vi "Main.vi"() -> ()   [LabVIEW 2013]
uses:
  <vilib>/Analysis/Matrix/Datatypes/RealMatrix.ctl
  Parts.ctl
  ROS/Code/SubVIs/BaxterSide.ctl
  ROS/Code/SubVIs/BaxterCamera.ctl
  Arm Globals.vi
  Prim/Fwd Kenimatics - array.vi
  Move/Move Axis.vi
  Move/Move XYZOAT.vi
  <vilib>/Analysis/Matrix/NI_Matrix.lvlib
panel:
  in  "To":string="Table"
  in  "From":string="Table"
  in  "Both?":bool
  in  "Post Side":bool
  in  "Side":T1=enum."right"
  in  "Go Via":bool
  in  "Increment":dbl=50.0
  in  "Offset":cluster{"x":dbl, "y":dbl, "a":dbl}={"x"=50.0, "y"=900.0, "a"=0.0}
  in  "Offset":cluster{"x":dbl, "y":dbl, "a":dbl}={"x"=50.0, "y"=900.0, "a"=0.0}
  in  "Put":bool
  in  "Locate Tray":bool
  in  "Part":T2 items=["Big_Gear", "Medium_Gear", "Small_Gear", "Bottom_Cover", "Top_Cover"]
  in  "Fetch":bool
  out "T":T3=[[0.016284994521607307, 0.9998576764567041, 0.0044074691186384496, -12.095922523672678], [0.9998670931969393, -0.01628143110047913, -0.0008431744914288715, -1019.3924117975101], [-0.0007712945830650122, 0.004420614427981981, -0.999989931585686, 240.25900755427352], [0.0, 0.0, 0.0, 1.0]] format="%.3f"
  out "picture":picture
  out "Range":u32=104
  in  "Speed":dbl=25.0
  in  "Shift":cluster{"x":dbl, "y":dbl, "a":dbl}={"x"=-110.0, "y"=-70.0, "a"=0.0}
  in  "Shift":bool
  in  "Go Safe":bool
  in  "Save Pic":bool
  in  "Image":bool
  in  "Gripper":bool caption="Open\n\n\n\nClose"
  in  "Hover Height":dbl=200.0
  in  "Hover":bool
  # "Y"
  # "X"
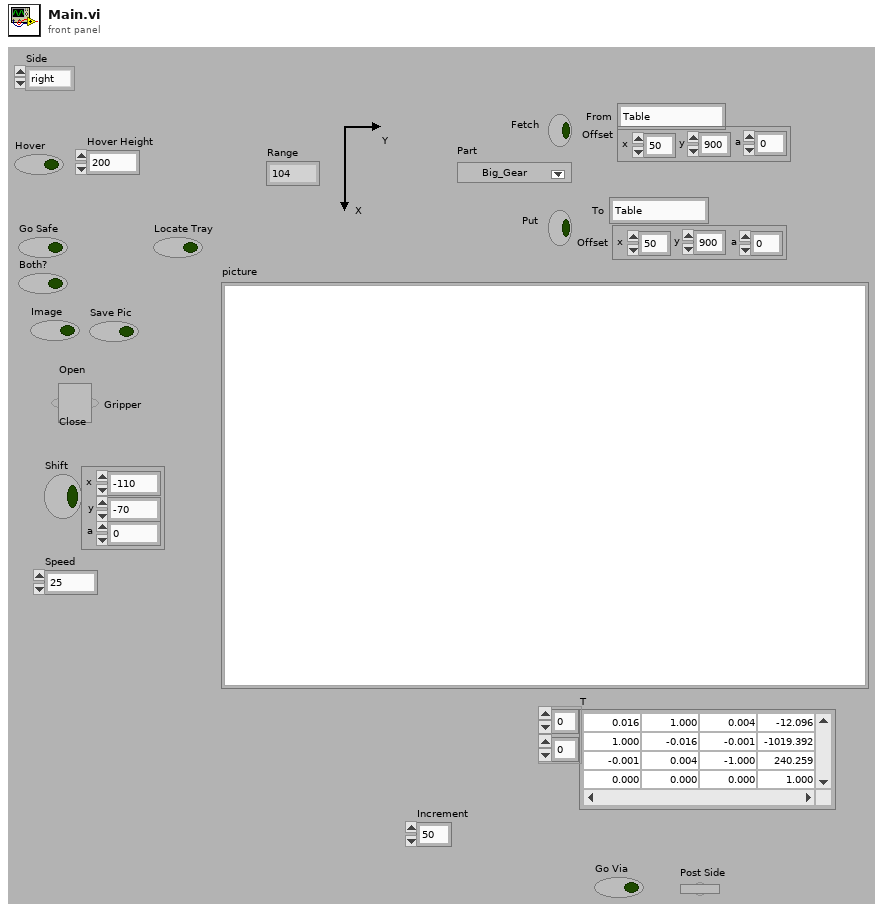
[diagram p1: front panel]
types:
  T1 = typedef "BaxterSide.ctl" = enum16{"left", "right"}
  T2 = typedef "Parts.ctl" = u16
  T3 = typedef "NI_Matrix.lvlib/RealMatrix.ctl" = dbl[][]
  T4 = typedef "BaxterCamera.ctl" = enum16{"left_hand_camera", "right_hand_camera", "head_camera"}
  T5 = cluster{"X":dbl, "Y":dbl, "Z":dbl, "Roll":dbl, "Pitch":dbl, "Yaw":dbl}
  T6 = typedef "imagedata.ctl" = cluster{"image type":i32, "image depth":i32, "image":u8[], "mask":u8[], "colors":u32[], "Rectangle":cluster{"left":i16, "top":i16, "right":i16, "bottom":i16}}
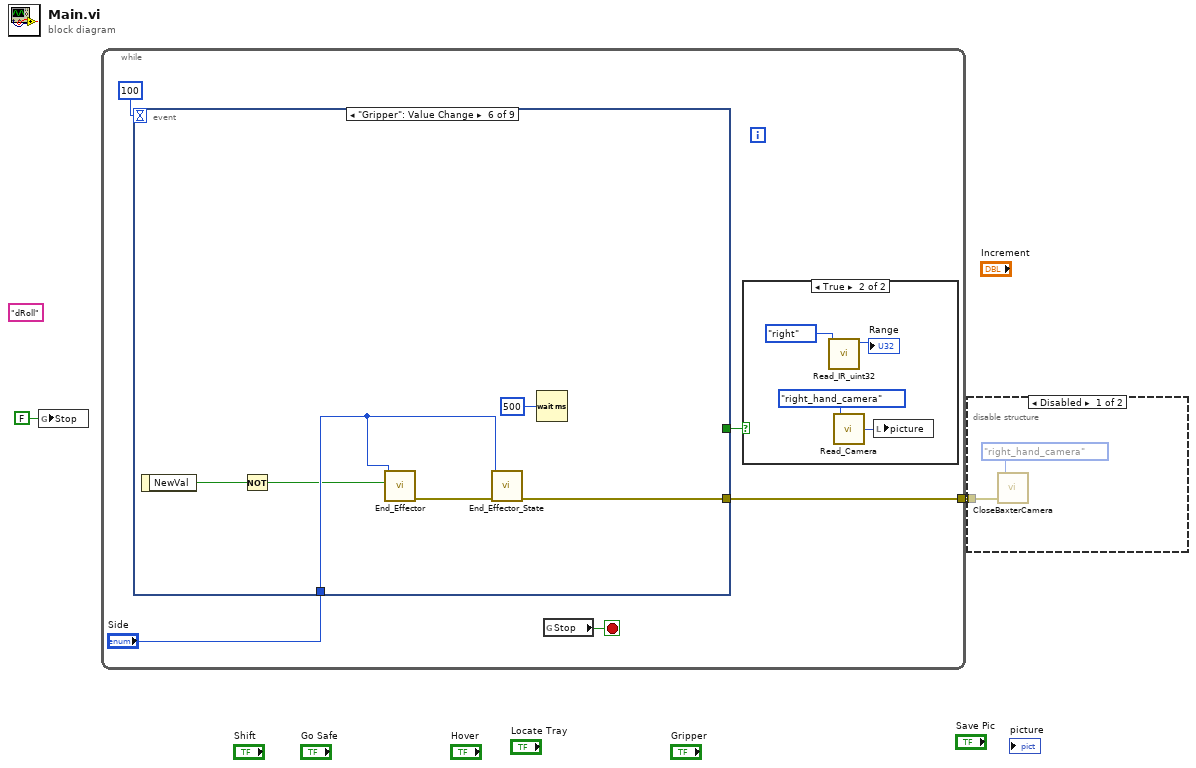
[diagram p0: block diagram]
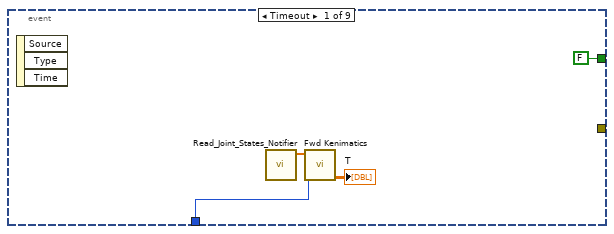
[diagram p4: hidden frame]
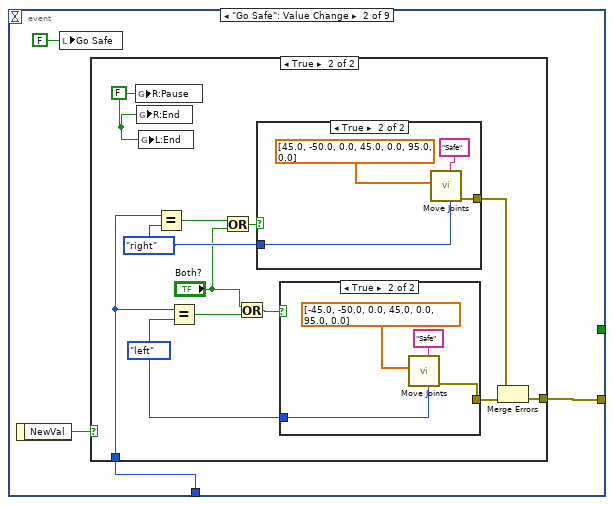
[diagram p5: hidden frame]
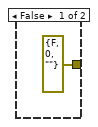
[diagram p6: hidden frame]
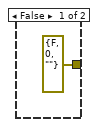
[diagram p7: hidden frame]
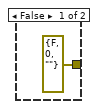
[diagram p8: hidden frame]
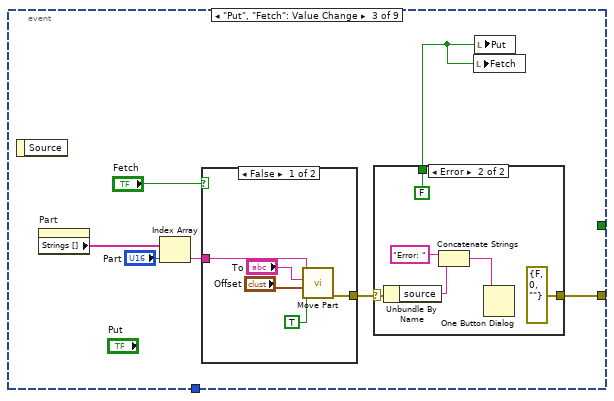
[diagram p9: hidden frame]
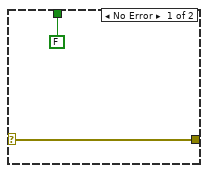
[diagram p10: hidden frame]
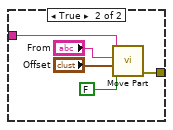
[diagram p11: hidden frame]
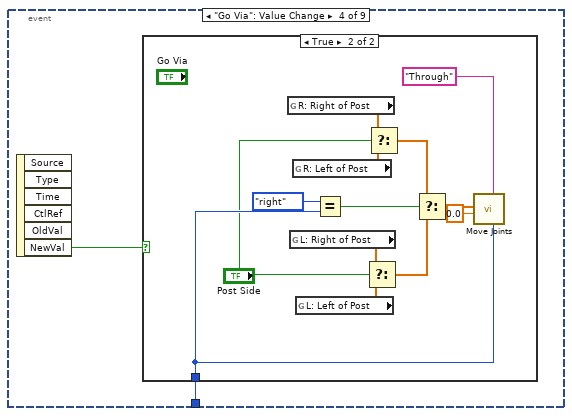
[diagram p12: hidden frame]
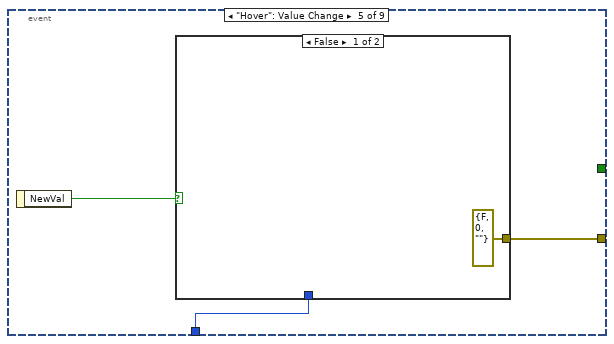
[diagram p14: hidden frame]
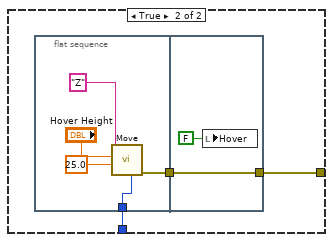
[diagram p15: hidden frame]
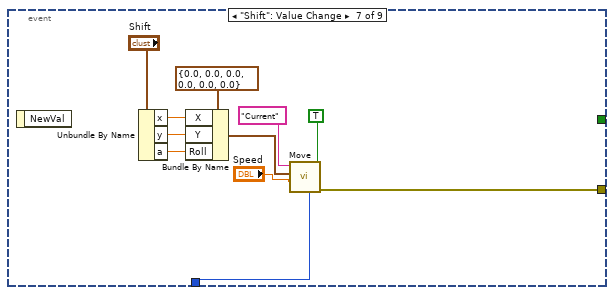
[diagram p16: hidden frame]
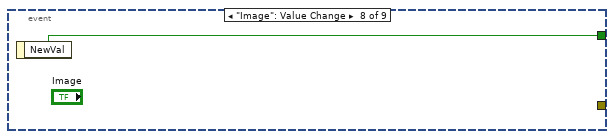
[diagram p17: hidden frame]
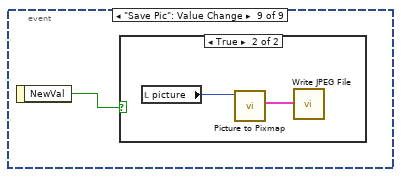
[diagram p18: hidden frame]
diagram:
  (unwired) "dRoll" ("Label")
  n1 = global write "Arm Globals.vi" "Stop"(FALSE ("Stop")) -> ()
  n2 = while {
    tunnel: [w6] -> w1
    stop <- w7 stop-if-true
    n3 = event shown="[5] \"Gripper\": Value Change" {
      selector: _ -> [_ _ _ _ _ _ _ _ _]
      dyn-events: _ -> [_ _ _ _ _ _ _ _ _]
      timeout: 100 -> [_ _ _ _ _ _ _ _ _]
      tunnel: [_ w18 w43 _ w84 w99 w113 _ _] -> w6
      tunnel: "Side" -> [w13 w16 _ w68 w83 w98 w103 _ _]
      tunnel: [FALSE ("NewVal") _ _ _ _ _ _ w114 _] -> w4
      event Timeout {
        n4 = event-data() -> ()  [unwired: 1 in, 3 out]
        n5 = call "Read_Joint_States_Notifier.vi"() -> ("Positions"=w14:dbl[])  [unwired: 7 in, 1 out]
        n6 = call-poly "Fwd Kenimatics.vi"("Side"=w13, "Joints"=w14) -> ("Matrix"=→"T":T3)  [unwired: 8 in, 1 out]
      }
      event "Go Safe": Value Change {
        n7 = event-data() -> ("NewVal"=w19:bool)  [unwired: 1 in]
        n8 = local write "Go Safe"(FALSE ("Go Safe")) -> ()
        n9 = case shown="True" w19 {
          tunnel: [errorcluster {"status"=FALSE, "code"=0, "source"=""} ("error IO") w32] -> w18
          tunnel: w16 -> [_ w28]
          frame False {
          }
          frame True {
            w27 = BaxterSide."left" ("x")
            w29 = BaxterSide."right" ("x")
            w21 = FALSE ("R:Pause")
            n10 = global write "Arm Globals.vi" "R:Pause"(w21) -> ()
            n11 = global write "Arm Globals.vi" "R:End"(w21) -> ()
            n12 = global write "Arm Globals.vi" "L:End"(w21) -> ()
            n13 = Equal?(x=w28, y=w29) -> (x = y?=w23:bool)
            n14 = Equal?(x=w28, y=w27) -> (x = y?=w24:bool)
            n15 = Or(x=w23, y="Both?") -> (x .or. y?=w26:bool)
            n16 = Or(x="Both?", y=w24) -> (x .or. y?=w25:bool)
            n17 = case shown="True" w26 {
              tunnel: w29 -> [_ w36]
              tunnel: [errorcluster {"status"=FALSE, "code"=0, "source"=""} ("error out") w35] -> w30
              frame False {
              }
              frame True {
                n18 = call "Move Joints.vi"("Side"=w36, "Label"="Safe", "Goal"=dbl[] [45.0, -50.0, 0.0, 45.0, 0.0, 95.0, 0.0] ("Joints")) -> ("error out"=w35:errorcluster)  [unwired: 7 in, 1 out]
              }
            }
            n19 = case shown="True" w25 {
              tunnel: [errorcluster {"status"=FALSE, "code"=0, "source"=""} ("error out") w40] -> w31
              tunnel: w27 -> [_ w39]
              frame False {
              }
              frame True {
                n20 = call "Move Joints.vi"("Side"=w39, "Label"="Safe", "Goal"=dbl[] [-45.0, -50.0, 0.0, 45.0, 0.0, 95.0, 0.0] ("Joints")) -> ("error out"=w40:errorcluster)  [unwired: 7 in, 1 out]
              }
            }
            n21 = Merge Errors(w30, w31) -> (w32:errorcluster)
          }
        }
      }
      event "Put", "Fetch": Value Change {
        n22 = event-data() -> ()  [unwired: 1 in, 1 out]
        n23 = property on="Part" class="Ring (strict)"() -> ("Strings []"=w47:string[])  [unwired: 2 in, 2 out]
        n24 = Index Array(array=w47, index="Part") -> (element=w48:string)
        n25 = case shown="False" "Fetch" {
          tunnel: [w62 w67] -> w45
          tunnel: w48 -> [w59 w64]
          frame False {
            n26 = call "Move Part.vi"("Place"=TRUE ("Place?"), "Offset"="Offset", "Location"="To", "Part Name"=w59) -> ("error out"=w62:errorcluster)  [unwired: 7 in]
          }
          frame True {
            n27 = call "Move Part.vi"("Place"=FALSE ("Place?"), "Offset"="Offset", "Location"="From", "Part Name"=w64) -> ("error out"=w67:errorcluster)  [unwired: 7 in]
          }
        }
        n28 = case shown="Error" w45 {
          selector: w45 -> [w50 w56]
          tunnel: [FALSE ("Compute Pose") FALSE ("Compute Pose")] -> w44
          tunnel: [w50 errorcluster {"status"=FALSE, "code"=0, "source"=""} ("error IO")] -> w43
          frame No Error {
          }
          frame Error {
            n29 = Unbundle By Name(w56) -> ("source"=w54:string)
            n30 = Concatenate Strings("Error: " ("string"), w54) -> (w53:string)
            n31 = One Button Dialog(message=w53) -> ()  [unwired: 1 in, 1 out]
          }
        }
        n32 = local write "Fetch"(w44) -> ()
        n33 = local write "Put"(w44) -> ()
      }
      event "Go Via": Value Change {
        n34 = event-data() -> ("NewVal"=w69:bool)  [unwired: 1 in, 5 out]
        n35 = case shown="True" w69 {
          tunnel: w68 -> [_ w77]
          frame False {
          }
          frame True {
            n36 = global read "Arm Globals.vi" "R: Right of Post"() -> (w70:dbl[])
            n37 = global read "Arm Globals.vi" "L: Right of Post"() -> (w75:dbl[])
            n38 = global read "Arm Globals.vi" "R: Left of Post"() -> (w72:dbl[])
            n39 = global read "Arm Globals.vi" "L: Left of Post"() -> (w74:dbl[])
            n40 = Equal?(x=BaxterSide."right", y=w77) -> (x = y?=w80:bool)
            n41 = Select(t=w75, s="Post Side", f=w74) -> (s? t:f=w76:dbl[])
            n42 = Select(t=w70, s="Post Side", f=w72) -> (s? t:f=w73:dbl[])
            n43 = Select(t=w73, s=w80, f=w76) -> (s? t:f=w78:dbl[])
            n44 = call "Move Joints.vi"("Side"=w77, "Label"="Through" ("format string"), "time"=0.0, "Goal"=w78) -> ()  [unwired: 6 in, 2 out]
          }
        }
      }
      event "Hover": Value Change {
        n45 = event-data() -> ("NewVal"=w85:bool)  [unwired: 1 in]
        n46 = case "Move to High Hover" shown="False" w85 {
          tunnel: [errorcluster {"status"=FALSE, "code"=0, "source"=""} ("error out") w89] -> w84
          tunnel: w83 -> [_ w88]
          frame False {
          }
          frame True {
            n47 = flat-sequence {
              tunnel: w88 -> [w90]
              tunnel: [w94] -> w87
              tunnel: [w96] -> w89
              tunnel: w87 -> [w96]
              frame #0 {
                n48 = call-poly "Move.vi"("Side"=w90, "Speed"=25.0, "Value"="Hover Height", "Location"="Z" ("Axis")) -> ("error out"=w94:errorcluster)  [unwired: 7 in]
              }
              frame #1 {
                n49 = local write "Hover"(FALSE ("Hover")) -> ()
              }
            }
          }
        }
      }
      event "Gripper": Value Change {
        n50 = event-data() -> ("NewVal"=w102:bool)  [unwired: 1 in]
        n51 = Not(x=w102) -> (.not. x?=w97:bool)
        n52 = call "End_Effector.vi"("Close"=w97, "Side"=w98) -> ("error out"=w100:errorcluster)  [unwired: 6 in]
        n53 = call "End_Effector_State.vi"("error in"=w100, "Side"=w98) -> ("error out"=w99:errorcluster)  [unwired: 4 in, 2 out]
        n54 = Wait (ms)(milliseconds to wait=u32 500) -> ()  [unwired: 1 out]
      }
      event "Shift": Value Change {
        n55 = event-data() -> ()  [unwired: 1 in, 1 out]
        n56 = Unbundle By Name("Shift") -> ("x"=w110:dbl, "y"=w109:dbl, "a"=w108:dbl)
        n57 = Bundle By Name(cluster=T5 {"X"=0.0, "Y"=0.0, "Z"=0.0, "Roll"=0.0, "Pitch"=0.0, "Yaw"=0.0} ("XYZOAT"), "X"=w110, "Y"=w109, "Roll"=w108) -> (w105:T5)
        n58 = call-poly "Move.vi"("Make Vertical"=TRUE, "Side"=w103, "Speed (mm/s)"="Speed", "XYZOAT"=w105, "Location"="Current") -> ("error out"=w113:errorcluster)  [unwired: 6 in]
      }
      event "Image": Value Change {
        n59 = event-data() -> ("NewVal"=w114:bool)  [unwired: 1 in]
      }
      event "Save Pic": Value Change {
        n60 = event-data() -> ("NewVal"=w115:bool)  [unwired: 1 in]
        n61 = case shown="True" w115 {
          frame False {
          }
          frame True {
            n62 = local read "picture"() -> (w117:picture)
            n63 = call <vilib>:"Picture to Pixmap.vi"("picture"=w117) -> ("image data"=w116:T6)  [unwired: 9 in, 1 out]
            n64 = call <vilib>:"Write JPEG File.vi"("image data"=w116) -> ()  [unwired: 9 in, 2 out]
          }
        }
      }
    }
    n65 = global read "Arm Globals.vi" "Stop"() -> (w7:bool)
    n66 = case shown="True" w4 {
      frame False {
      }
      frame True {
        n67 = call "Read_IR_uint32.vi"("Side"=BaxterSide."right") -> ("Range"=→"Range":u32)  [unwired: 4 in, 3 out]
        n68 = call "Read_Camera.vi"("Camera"=BaxterCamera."right_hand_camera") -> ("picture"=w11:picture)  [unwired: 4 in, 2 out]
        n69 = local write "picture"(w11) -> ()
      }
    }
  }
  n70 = disable-structure shown="Disabled" {
    disable-tunnel: w1 -> [w119 _]
    frame Disabled {
      n71 = call "CloseBaxterCamera.vi"("error in"=w119, "Camera"=BaxterCamera."right_hand_camera") -> ()  [unwired: 1 in, 3 out]
    }
    frame Enabled {
    }
  }
